vi "Zigmar_Zigmap.vi"(10 "Paso":dbl, 11 "Tiempo":dbl) -> (1 "Xdrp":dbl[](array[numeric]), 2 "Phir":dbl[](array[numeric]), 3 "Ydr":dbl[](array[numeric]), 4 "Ydrp":dbl[](array[numeric]), 5 "Xdr":dbl[](array[numeric]), 6 "Phirp":dbl[](array[numeric]))   [LabVIEW 2011]
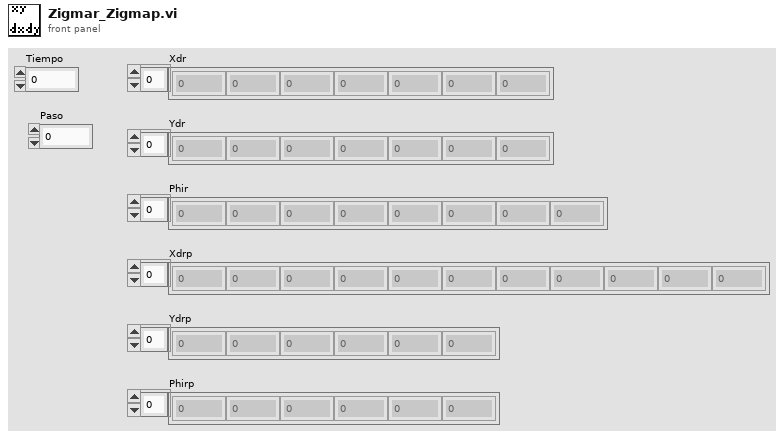
[diagram p1: front panel]
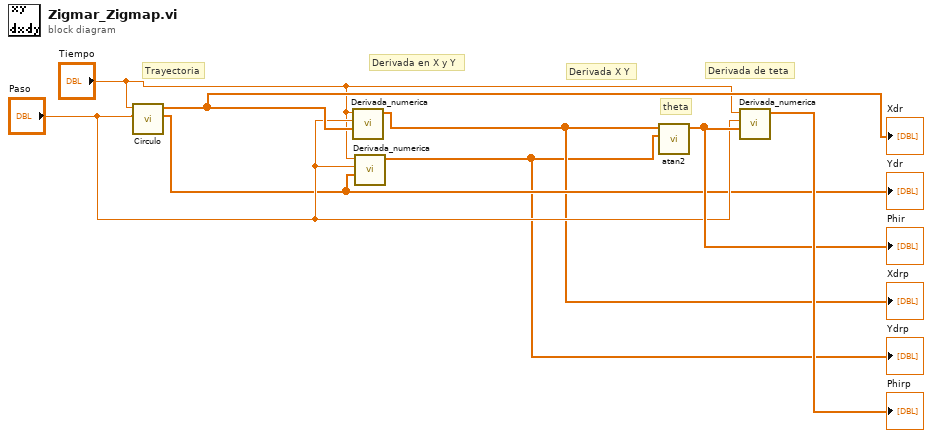
[diagram p0: block diagram]
diagram:
  # "Derivada en X y Y"
  # "Derivada de teta"
  # "theta"
  # "Derivada X Y"
  # "Trayectoria"
  n1 = call "Circulo.vi"("Paso"="Paso", "Tiempo"="Tiempo") -> ("Y"=w4:dbl[], "X"=w6:dbl[])  [unwired: 8 in]
  "Ydr" <- w4
  "Xdr" <- w6
  n2 = call "Derivada_numerica.vi"("Funcion"=w6, "Paso"="Paso", "Tiempo"="Tiempo") -> ("Derivada"=w2:dbl[])  [unwired: 8 in]
  "Xdrp" <- w2
  n3 = call "Derivada_numerica.vi"("Funcion"=w4, "Paso"="Paso", "Tiempo"="Tiempo") -> ("Derivada"=w1:dbl[])  [unwired: 8 in]
  "Ydrp" <- w1
  n4 = call "atan2.vi"("Y"=w1, "X"=w2) -> ("atan2"=w7:dbl[])  [unwired: 9 in]
  "Phir" <- w7
  n5 = call "Derivada_numerica.vi"("Funcion"=w7, "Paso"="Paso", "Tiempo"="Tiempo") -> ("Derivada"=→"Phirp":dbl[])  [unwired: 8 in]
